vi "s3path.get.vi"(8 "error in (no error)":errorcluster, 11 "s3path in":refnum<class "s3path.lvclass">) -> (0 "error out":errorcluster, 2 "s3path":string, 3 "s3path out":refnum<class "s3path.lvclass">)   [LabVIEW 2020, in "nominal types.lvlib" / "timestampManifest.lvlib" / "s3path.lvclass"]
uses:
  s3path.lvclass
  s3path.lvclass/s3path.ctl
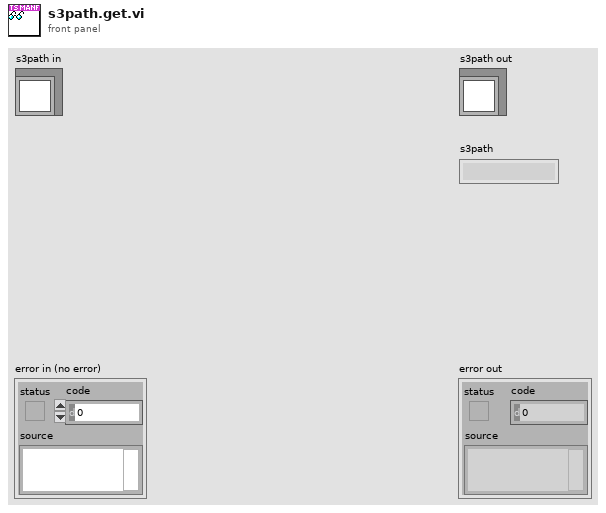
[diagram p1: front panel]
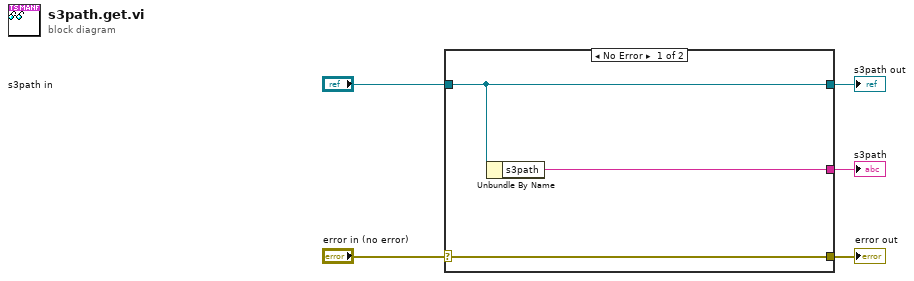
[diagram p0: block diagram]
diagram:
  n1 = case shown="No Error" "error in (no error)" {
    selector: "error in (no error)" -> [w8 w9]
    tunnel: [w8 w9] -> w4
    tunnel: [w7 w10] -> w2
    tunnel: "s3path in" -> [w7 w10]
    tunnel: [w6 _] -> w1
    frame No Error {
      n2 = Unbundle By Name(w7) -> ("s3path"=w6:string)
    }
    frame Error {
    }
  }
  "error out" <- w4
  "s3path out" <- w2
  "s3path" <- w1
